vi "Folder Sync.vi"(7 "Copy(default)/Move":enum16{"Copy", "Move"}(ring), 8 "error in (no error)":errorcluster, 9 "Exclusion File List":string[](array[string]), 10 "Destination Folder (To be modified)":path, 11 "Source Folder":path) -> (0 "error out":errorcluster, 3 "List of Files Copied/Moved":string[](array[string]))   [LabVIEW 2012]
doc: "SciScan 1.2 160622"
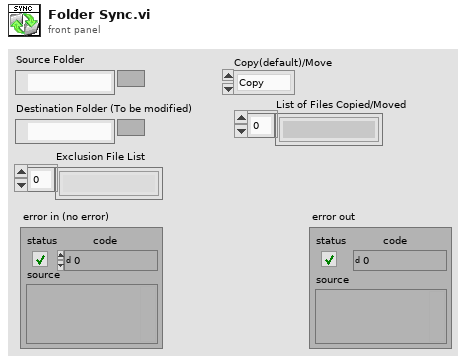
[diagram p1: front panel]
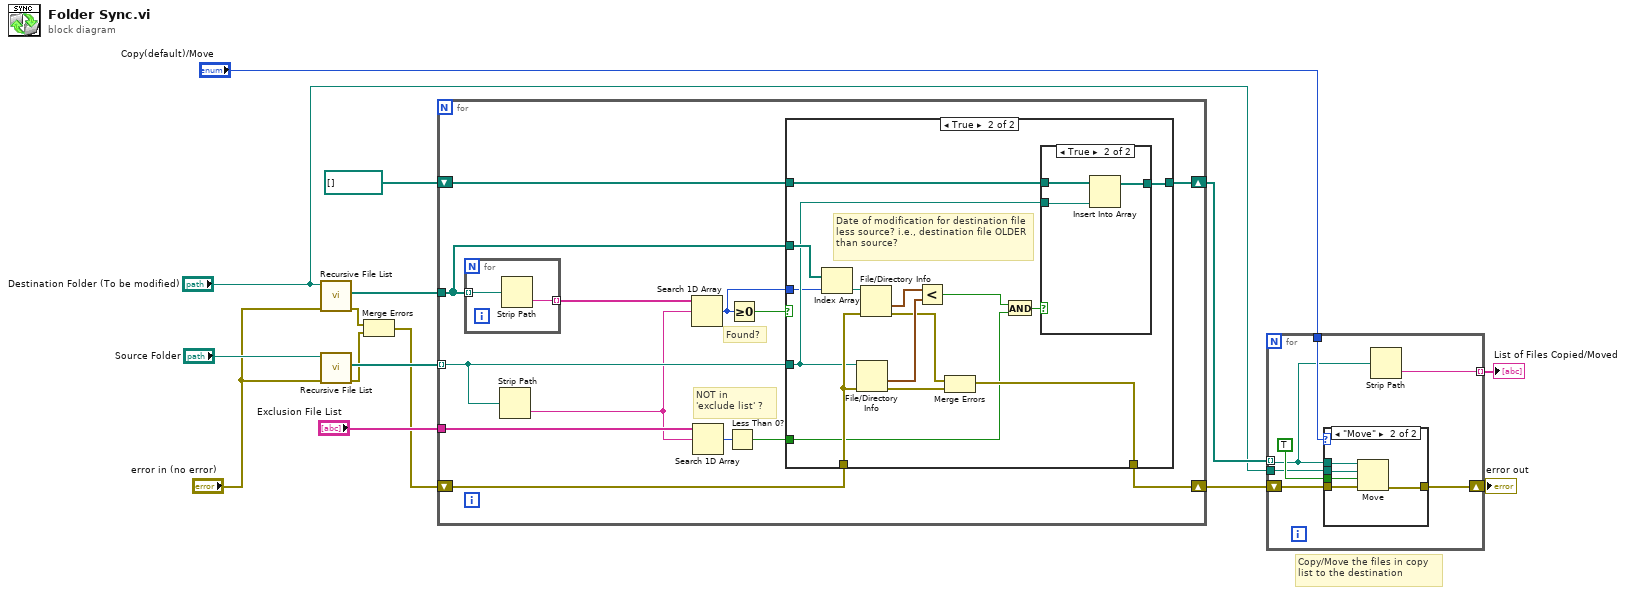
[diagram p0: block diagram]
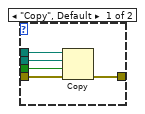
[diagram p2: hidden frame]
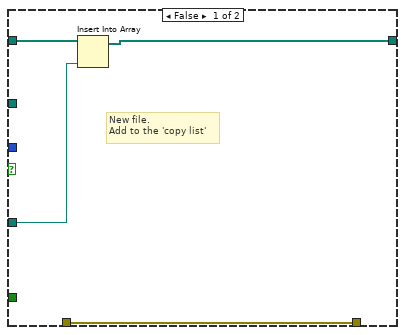
[diagram p3: hidden frame]
diagram:
  # "Copy/Move the files in copy list to the destination"
  n1 = call <vilib>:"Recursive File List.vi"("error in (no error)"="error in (no error)", "Folder Path"="Destination Folder (To be modified)") -> ("error out"=w3:errorcluster, "All Files in Dir"=w13:path[])  [unwired: 5 in, 3 out]
  n2 = call <vilib>:"Recursive File List.vi"("error in (no error)"="error in (no error)", "Folder Path"="Source Folder") -> ("error out"=w2:errorcluster, "All Files in Dir"=w14:path[])  [unwired: 5 in, 3 out]
  n3 = Merge Errors(w3, w2) -> (w1:errorcluster)
  n4 = for {
    shift-right: [w25] -> w10
    shift-left: path[] [] -> [w26]
    tunnel: w14 -> [w23] mode=indexing
    tunnel: w13 -> [w22]
    tunnel: "Exclusion File List" -> [w19]
    shift-right: [w20] -> w8
    shift-left: w1 -> [w21]
    # "NOT in \n'exclude list' ?"
    # "Found?"
    n5 = for {
      tunnel: w22 -> [w30] mode=indexing
      tunnel: [w29] -> w24 mode=indexing
      n6 = Strip Path(path=w30) -> (name=w29:string)  [unwired: 1 out]
    }
    n7 = Strip Path(path=w23) -> (name=w18:string)  [unwired: 1 out]
    n8 = Search 1D Array(1D array=w24, element=w18) -> (index of element=w27:i32)  [unwired: 1 in]
    n9 = Search 1D Array(1D array=w19, element=w18) -> (index of element=w17:i32)  [unwired: 1 in]
    n10 = Less Than 0?(x=w17) -> (x < 0?=w16:bool)
    n11 = Greater Or Equal To 0?(x=w27) -> (x >= 0?=w28:bool)
    n12 = case shown="True" w28 {
      tunnel: w26 -> [w34 w46]
      tunnel: w23 -> [w32 w45]
      tunnel: [w33 w43] -> w25
      tunnel: w27 -> [_ w44]
      tunnel: w22 -> [_ w49]
      tunnel: w21 -> [w31 w48]
      tunnel: [w31 w47] -> w20
      tunnel: w16 -> [_ w35]
      frame False {
        # "New file.\nAdd to the 'copy list'"
        n13 = Insert Into Array(array=w34, new element=w32) -> (w33:path[])  [unwired: 1 in]
      }
      frame True {
        # "Date of modification for destination file less source? i.e., destination file OLDER than source?"
        n14 = Index Array(array=w49, index=w44) -> (element=w42:path)
        n15 = File/Directory Info(path=w45, error in=w48) -> (last mod=w40:timestamp, error out=w39:errorcluster)  [unwired: 5 out]
        n16 = File/Directory Info(path=w42, error in=w48) -> (last mod=w41:timestamp, error out=w38:errorcluster)  [unwired: 5 out]
        n17 = Less?(x=w41, y=w40) -> (x < y?=w37:bool)
        n18 = Merge Errors(w38, w39) -> (w47:errorcluster)
        n19 = And(x=w37, y=w35) -> (x .and. y?=w36:bool)
        n20 = case shown="True" w36 {
          tunnel: w46 -> [w50 w53]
          tunnel: w45 -> [_ w52]
          tunnel: [w50 w51] -> w43
          frame False {
          }
          frame True {
            n21 = Insert Into Array(array=w53, new element=w52) -> (w51:path[])  [unwired: 1 in]
          }
        }
      }
    }
  }
  n22 = for {
    tunnel: w10 -> [w55] mode=indexing
    tunnel: "Destination Folder (To be modified)" -> [w59]
    shift-right: [w57] -> w7
    shift-left: w8 -> [w58]
    tunnel: "Copy(default)/Move" -> [w56]
    tunnel: [w54] -> w5 mode=indexing
    n23 = case shown="\"Move\"" w56 {
      tunnel: TRUE ("overwrite (F)") -> [w65 w68]
      tunnel: w55 -> [w64 w67]
      tunnel: w59 -> [w63 w66]
      tunnel: w58 -> [w62 w70]
      tunnel: [w61 w69] -> w57
      frame "Copy", Default {
        n24 = Copy(8:w62, 9:w65, 10:w63, 11:w64) -> (0:w61:errorcluster)  [unwired: 1 in, 2 out]
      }
      frame "Move" {
        n25 = Move(source path=w67, error in=w70, 9:w68, 10:w66) -> (error out=w69:errorcluster)  [unwired: 1 in, 2 out]
      }
    }
    n26 = Strip Path(path=w55) -> (name=w54:string)  [unwired: 1 out]
  }
  "error out" <- w7
  "List of Files Copied/Moved" <- w5
